vi "singleOut.vi"() -> ()   [LabVIEW 2016]
panel:
  in  "HIFU in":refnum<visa-resource-name>
  in  "channel":u8=1
  in  "cycles":dbl=10.0
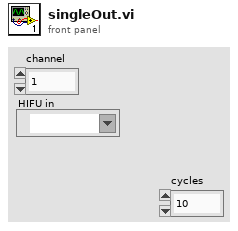
[diagram p1: front panel]
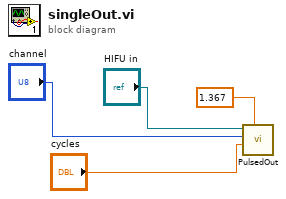
[diagram p0: block diagram]
diagram:
  n1 = call "PulsedOut.vi"("HIFU UART in"="HIFU in", "Channel"="channel", "Cycles"="cycles", "frequency (MHz)"=1.367) -> ()  [unwired: 1 in, 3 out]
